vi "Dir Factory.vi"(8 "error in (no error)":errorcluster, 11 "Commands":string[](array[string])) -> (0 "error out":errorcluster, 3 "dir out":refnum<class "dir.lvclass">)   [LabVIEW 2023, in "d7.lvlib" / "dir.lvclass"]
uses:
  dir.lvclass
  C:/Projects/lv2023-advent-of-code-2023/d7/node/node.lvclass
  C:/Projects/lv2023-advent-of-code-2023/d7/INode/INode.lvclass
  file/file.lvclass
  node/node.lvclass
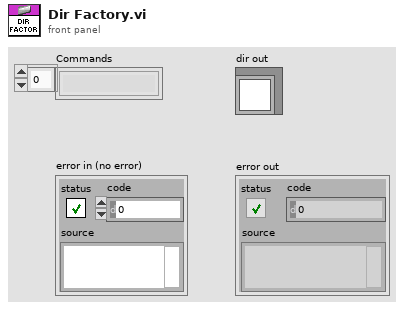
[diagram p1: front panel]
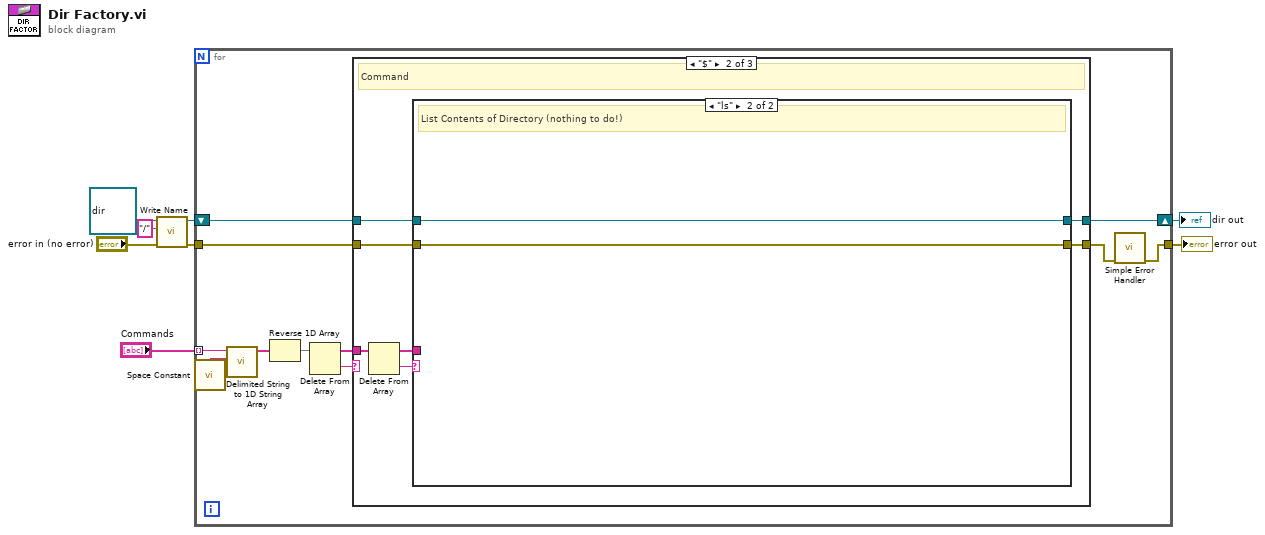
[diagram p0: block diagram]
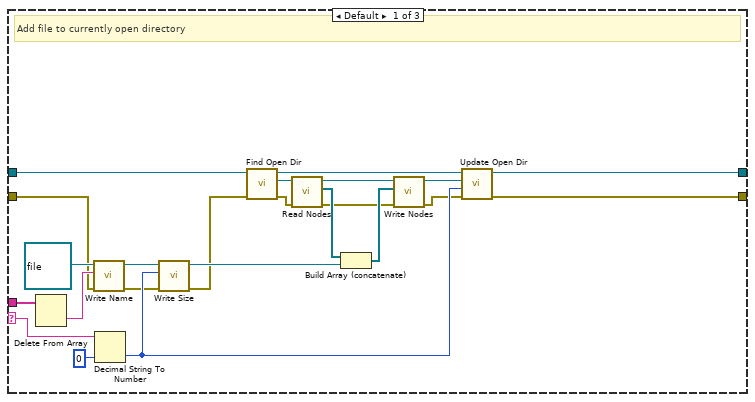
[diagram p2: hidden frame]
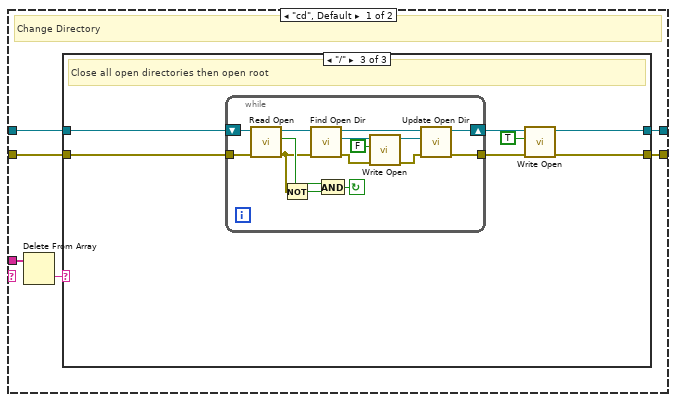
[diagram p3: hidden frame]
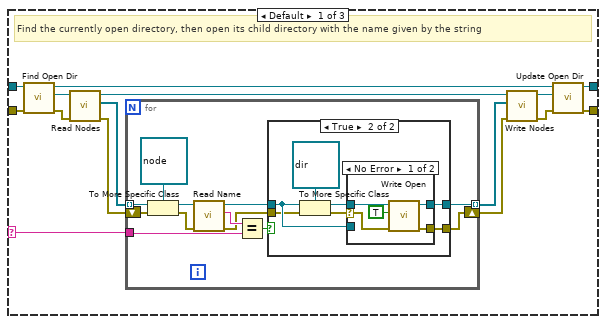
[diagram p4: hidden frame]
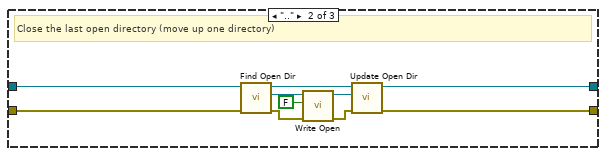
[diagram p7: hidden frame]
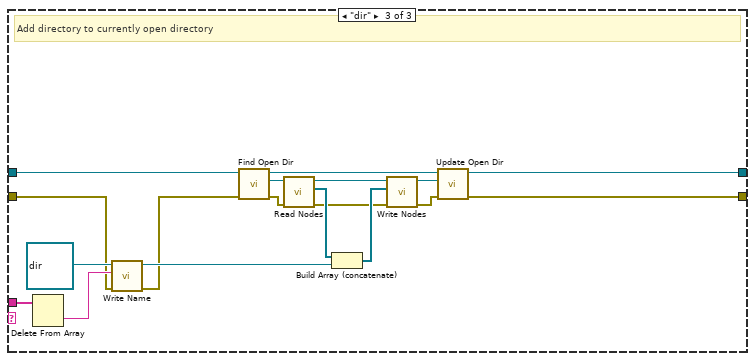
[diagram p8: hidden frame]
diagram:
  n1 = call-dynamic "Write Name.vi"("error in (no error)"="error in (no error)", "Name"="/", "node in"=refnum<class "dir.lvclass"> refnum ("d7.lvlib:dir.lvclass")) -> ("error out"=w3:errorcluster, "node out"=w6:refnum<class "dir.lvclass">)  [unwired: 7 in]
  n2 = for {
    tunnel: "Commands" -> [w19] mode=indexing
    shift-right: [w13] -> w7
    shift-left: w6 -> [w15]
    tunnel: w3 -> [w11]
    tunnel: [w9] -> w2
    n3 = call <vilib>:"Space Constant.vi"() -> ("String"=w18:string)
    n4 = call <vilib>:"Delimited String to 1D String Array.vi"("delimiter"=w18, "delimited string"=w19) -> ("string array"=w17:string[])  [unwired: 9 in]
    n5 = Reverse 1D Array(array=w17) -> (reversed array=w12:string[])
    n6 = Delete From Array(array=w12) -> (deleted portion=w16:string, array with subset deleted=w14:string[])  [unwired: 2 in]
    n7 = case shown="\"$\"" w16 {
      selector: w16 -> [w33 _ _]
      tunnel: w15 -> [w32 w49 w142]
      tunnel: w14 -> [w39 w47 w149]
      tunnel: [w28 w48 w141] -> w13
      tunnel: w11 -> [w20 w44 w133]
      tunnel: [w23 w43 w135] -> w10
      frame Default {
        # "Add file to currently open directory"
        n8 = Delete From Array(array=w39) -> (deleted portion=w38:string)  [unwired: 2 in, 1 out]
        n9 = call-dynamic "Write Name.vi"("error in (no error)"=w20, "Name"=w38, "node in"=refnum<class "file.lvclass"> refnum ("d7.lvlib:file.lvclass")) -> ("error out"=w22:errorcluster, "node out"=w40:refnum<class "file.lvclass">)  [unwired: 7 in]
        n10 = Decimal String To Number(string=w33, default (0L)=i64 0 ("default (0 I32)")) -> (number=w27:i64)  [unwired: 1 in, 1 out]
        n11 = call-dynamic "Write Size.vi"("error in (no error)"=w22, "Size"=w27, "file in"=w40) -> ("error out"=w21:errorcluster, "file out"=w36:refnum<class "file.lvclass">)  [unwired: 7 in]
        n12 = call "Find Open Dir.vi"("error in (no error)"=w21, "dir in"=w32) -> ("error out"=w26:errorcluster, "open dir"=w31:refnum<class "dir.lvclass">, "dir out"=w30:refnum<class "dir.lvclass">)  [unwired: 7 in]
        n13 = call-dynamic "Read Nodes.vi"("error in (no error)"=w26, "dir in"=w31) -> ("error out"=w25:errorcluster, "Nodes"=w37:refnum<class "INode.lvclass">[], "dir out"=w42:refnum<class "dir.lvclass">)  [unwired: 7 in]
        n14 = Build Array (concatenate)(w37, w36) -> (w35:refnum<class "INode.lvclass">[])
        n15 = call-dynamic "Write Nodes.vi"("error in (no error)"=w25, "Nodes"=w35, "dir in"=w42) -> ("error out"=w24:errorcluster, "dir out"=w29:refnum<class "dir.lvclass">)  [unwired: 7 in]
        n16 = call "Update Open Dir.vi"("error in (no error)"=w24, "Size to Add"=w27, "open dir"=w29, "dir in"=w30) -> ("error out"=w23:errorcluster, "dir out"=w28:refnum<class "dir.lvclass">)  [unwired: 6 in]
      }
      frame "$" {
        # "Command"
        n17 = Delete From Array(array=w47) -> (deleted portion=w46:string, array with subset deleted=w45:string[])  [unwired: 2 in]
        n18 = case shown="\"ls\"" w46 {
          tunnel: w49 -> [w55 w132]
          tunnel: [w54 w132] -> w48
          tunnel: w45 -> [w53 _]
          tunnel: w44 -> [w51 w131]
          tunnel: [w50 w131] -> w43
          frame "cd", Default {
            # "Change Directory"
            n19 = Delete From Array(array=w53) -> (deleted portion=w52:string)  [unwired: 2 in, 1 out]
            n20 = case shown="\"/\"" w52 {
              selector: w52 -> [w63 _ _]
              tunnel: w55 -> [w66 w107 w115]
              tunnel: [w65 w106 w113] -> w54
              tunnel: w51 -> [w61 w102 w111]
              tunnel: [w58 w99 w109] -> w50
              frame Default {
                # "Find the currently open directory, then open its child directory with the name given by the string"
                n21 = call "Find Open Dir.vi"("error in (no error)"=w61, "dir in"=w66) -> ("error out"=w60:errorcluster, "open dir"=w69:refnum<class "dir.lvclass">, "dir out"=w68:refnum<class "dir.lvclass">)  [unwired: 7 in]
                n22 = call-dynamic "Read Nodes.vi"("error in (no error)"=w60, "dir in"=w69) -> ("error out"=w56:errorcluster, "Nodes"=w64:refnum<class "INode.lvclass">[], "dir out"=w70:refnum<class "dir.lvclass">)  [unwired: 7 in]
                n23 = for {
                  tunnel: w64 -> [w82] mode=indexing
                  tunnel: w63 -> [w79]
                  tunnel: [w78] -> w62 mode=indexing
                  shift-right: [w74] -> w57
                  shift-left: w56 -> [w73]
                  n24 = To More Specific Class(target class=refnum<class "node.lvclass"> refnum ("node out"), reference=w82, error in=w73) -> (specific class reference=w81:refnum<class "node.lvclass">, error out=w72:errorcluster)
                  n25 = call-dynamic "Read Name.vi"("error in (no error)"=w72, "node in"=w81) -> ("error out"=w71:errorcluster, "Name"=w80:string, "node out"=w77:refnum<class "node.lvclass">)  [unwired: 7 in]
                  n26 = Equal?(x=w80, y=w79) -> (x = y?=w76:bool)
                  n27 = case shown="True" w76 {
                    tunnel: [w84 w91] -> w78
                    tunnel: w77 -> [w84 w87]
                    tunnel: [w83 w86] -> w74
                    tunnel: w71 -> [w83 w85]
                    frame False {
                    }
                    frame True {
                      n28 = To More Specific Class(target class=refnum<class "dir.lvclass"> refnum ("dir out"), reference=w87, error in=w85) -> (specific class reference=w90:refnum<class "dir.lvclass">, error out=w88:errorcluster)
                      n29 = case shown="No Error" w88 {
                        selector: w88 -> [w92 w97]
                        tunnel: [w96 w98] -> w91
                        tunnel: w90 -> [w95 _]
                        tunnel: w87 -> [_ w98]
                        tunnel: [w93 w97] -> w86
                        frame No Error {
                          n30 = call-dynamic "Write Open.vi"("error in (no error)"=w92, "Open"=TRUE, "dir in"=w95) -> ("error out"=w93:errorcluster, "dir out"=w96:refnum<class "dir.lvclass">)  [unwired: 7 in]
                        }
                        frame Error {
                        }
                      }
                    }
                  }
                }
                n31 = call-dynamic "Write Nodes.vi"("error in (no error)"=w57, "Nodes"=w62, "dir in"=w70) -> ("error out"=w59:errorcluster, "dir out"=w67:refnum<class "dir.lvclass">)  [unwired: 7 in]
                n32 = call "Update Open Dir.vi"("error in (no error)"=w59, "open dir"=w67, "dir in"=w68) -> ("error out"=w58:errorcluster, "dir out"=w65:refnum<class "dir.lvclass">)  [unwired: 7 in]
              }
              frame ".." {
                # "Close the last open directory (move up one directory)"
                n33 = call "Find Open Dir.vi"("error in (no error)"=w102, "dir in"=w107) -> ("error out"=w101:errorcluster, "open dir"=w105:refnum<class "dir.lvclass">, "dir out"=w108:refnum<class "dir.lvclass">)  [unwired: 7 in]
                n34 = call-dynamic "Write Open.vi"("error in (no error)"=w101, "Open"=FALSE, "dir in"=w105) -> ("error out"=w100:errorcluster, "dir out"=w104:refnum<class "dir.lvclass">)  [unwired: 7 in]
                n35 = call "Update Open Dir.vi"("error in (no error)"=w100, "open dir"=w104, "dir in"=w108) -> ("error out"=w99:errorcluster, "dir out"=w106:refnum<class "dir.lvclass">)  [unwired: 7 in]
              }
              frame "/" {
                # "Close all open directories then open root"
                n36 = while {
                  shift-right: [w124] -> w114
                  shift-left: w115 -> [w125]
                  tunnel: w111 -> [w123]
                  tunnel: [w120] -> w110
                  stop <- w118 continue-if-true
                  n37 = call-dynamic "Read Open.vi"("error in (no error)"=w123, "dir in"=w125) -> ("error out"=w117:errorcluster, "Open"=w119:bool, "dir out"=w126:refnum<class "dir.lvclass">)  [unwired: 7 in]
                  n38 = Not(x=w117) -> (.not. x?=w116:bool)
                  n39 = call "Find Open Dir.vi"("error in (no error)"=w117, "dir in"=w126) -> ("error out"=w122:errorcluster, "open dir"=w130:refnum<class "dir.lvclass">, "dir out"=w128:refnum<class "dir.lvclass">)  [unwired: 7 in]
                  n40 = And(x=w119, y=w116) -> (x .and. y?=w118:bool)
                  n41 = call-dynamic "Write Open.vi"("error in (no error)"=w122, "Open"=FALSE, "dir in"=w130) -> ("error out"=w121:errorcluster, "dir out"=w127:refnum<class "dir.lvclass">)  [unwired: 7 in]
                  n42 = call "Update Open Dir.vi"("error in (no error)"=w121, "open dir"=w127, "dir in"=w128) -> ("error out"=w120:errorcluster, "dir out"=w124:refnum<class "dir.lvclass">)  [unwired: 7 in]
                }
                n43 = call-dynamic "Write Open.vi"("error in (no error)"=w110, "Open"=TRUE, "dir in"=w114) -> ("error out"=w109:errorcluster, "dir out"=w113:refnum<class "dir.lvclass">)  [unwired: 7 in]
              }
            }
          }
          frame "ls" {
            # "List Contents of Directory (nothing to do!)"
          }
        }
      }
      frame "dir" {
        # "Add directory to currently open directory"
        n44 = Delete From Array(array=w149) -> (deleted portion=w148:string)  [unwired: 2 in, 1 out]
        n45 = call-dynamic "Write Name.vi"("error in (no error)"=w133, "Name"=w148, "node in"=refnum<class "dir.lvclass"> refnum ("d7.lvlib:dir.lvclass")) -> ("error out"=w134:errorcluster, "node out"=w139:refnum<class "dir.lvclass">)  [unwired: 7 in]
        n46 = call "Find Open Dir.vi"("error in (no error)"=w134, "dir in"=w142) -> ("error out"=w138:errorcluster, "open dir"=w145:refnum<class "dir.lvclass">, "dir out"=w144:refnum<class "dir.lvclass">)  [unwired: 7 in]
        n47 = call-dynamic "Read Nodes.vi"("error in (no error)"=w138, "dir in"=w145) -> ("error out"=w137:errorcluster, "Nodes"=w140:refnum<class "INode.lvclass">[], "dir out"=w147:refnum<class "dir.lvclass">)  [unwired: 7 in]
        n48 = Build Array (concatenate)(w140, w139) -> (w146:refnum<class "INode.lvclass">[])
        n49 = call-dynamic "Write Nodes.vi"("error in (no error)"=w137, "Nodes"=w146, "dir in"=w147) -> ("error out"=w136:errorcluster, "dir out"=w143:refnum<class "dir.lvclass">)  [unwired: 7 in]
        n50 = call "Update Open Dir.vi"("error in (no error)"=w136, "open dir"=w143, "dir in"=w144) -> ("error out"=w135:errorcluster, "dir out"=w141:refnum<class "dir.lvclass">)  [unwired: 7 in]
      }
    }
    n51 = call <vilib>:"Simple Error Handler.vi"("error in (no error)"=w10) -> ("error out"=w9:errorcluster)  [unwired: 4 in, 4 out]
  }
  "dir out" <- w7
  "error out" <- w2
